vi "GetAttributeViString.vi"(8 "error in (no error)":errorcluster {"code" format="%.0x"}, 9 "AttributeID":u32(ring)=1150162 items=["CHANNEL_MEASUREMENT_NAME"=1150162, "DRIVER_SETUP"=1050007, "GUIDED_CALIBRATION_CALIBRATION_STEP_DESCRIPTION"=1150154, "INSTRUMENT_FIRMWARE_REVISION"=1050510, "INSTRUMENT_MANUFACTURER"=1050511, "INSTRUMENT_MODEL"=1050512, "IO_RESOURCE_DESCRIPTOR"=1050304, "LOGICAL_NAME"=1050305, "MODEL_NUMBER"=1150169, "SPECIFIC_DRIVER_DESCRIPTION"=1050514, "SPECIFIC_DRIVER_REVISION"=1050551, "SPECIFIC_DRIVER_VENDOR"=1050513, "SUPPORTED_INSTRUMENT_MODELS"=1050327, "SYSTEM_SERIAL_NUMBER"=1150039, "WINDOW_TITLE"=1150131], 10 "RepCapIdentifier":string, 11 "instrument handle":refnum<k15>) -> (0 "error out":errorcluster {"code" format="%.0x"}, 2 "AttributeValue":string, 3 "instrument handle out":refnum<k15>)   [LabVIEW 2014, in "Agilent NA.lvlib"]
doc: "Gets a String attribute from the instrument driver.\nThe following Attributes are supported:\n\nCHANNEL_MEASUREMENT_NAME\nDRIVER_SETUP\nGUIDED_CALIBRATION_CALIBRATION_STEP_DESCRIPTION\nINSTRUMENT_FIRMWARE_REVISION\nINSTRUMENT_MANUFACTURER\nINSTRUMENT_MODEL\nIO_RESOURCE_DESCRIPTOR\nLOGICAL_NAME\nMODEL_NUMBER\nSPECIFIC_DRIVER_DESCRIPTION\nSPECIFIC_DRIVER_REVISION\nSPECIFIC_DRIVER_VENDOR\nSUPPORTED_INSTRUMENT_MODELS\nSYSTEM_SERIAL_NUMBER\nWINDOW_TITLE"
uses:
  Agilent NA.lvlib
  AgNA.dll
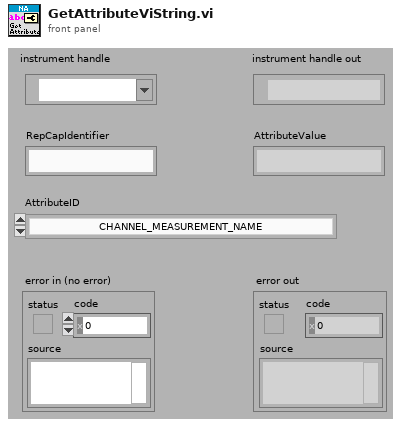
[diagram p1: front panel]
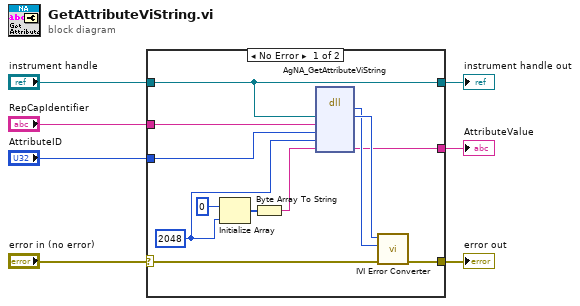
[diagram p0: block diagram]
diagram:
  n1 = case shown="No Error" "error in (no error)" {
    selector: "error in (no error)" -> [w17 w21]
    tunnel: [w16 w21] -> w7
    tunnel: "RepCapIdentifier" -> [w15 _]
    tunnel: "AttributeID" -> [w14 _]
    tunnel: [w10 _] -> w3
    tunnel: [w9 w20] -> w2
    tunnel: "instrument handle" -> [w9 w20]
    frame No Error {
      w8 = 2048 ("dimension size")
      n2 = Initialize Array(u8 0 ("element"), w8) -> (w12:u8[])
      n3 = Byte Array To String(unsigned byte array=w12) -> (string=w13:string)
      n4 = dll-call lib="AgNA**.dll" fn="AgNA_GetAttributeViString"("Vi"=w9, "RepCapIdentifier"=w15, "AttributeID"=w14, "AttributeValueBufferSize"=w8, "AttributeValue"=w13) -> ("return type"=w18:i32, "Vi"=w19:u32, "AttributeValue"=w10:string)  [unwired: 6 in, 2 out]
      n5 = call "IVI Error Converter.vi"("error in (no error)"=w17, "IVI error code (0)"=w18, "instrument handle"=w19) -> ("error out"=w16:errorcluster)  [unwired: 7 in, 1 out]
    }
    frame Error {
    }
  }
  "error out" <- w7
  "instrument handle out" <- w2
  "AttributeValue" <- w3
